vi "Signal_output_DAQ.vi"() -> ()   [LabVIEW 2013]
doc: "This example demonstrates how to continuously re-generate analog output data from a buffer in your computer's memory.\n\nRefer to your device documentation for pinouts and hardware capabilities."
uses:
  <vilib>/Utility/error.llb/DialogType.ctl
  <vilib>/DAQmx/write.llb/DAQmx Write (Analog 1D Wfm NChan NSamp).vi
  <vilib>/DAQmx/create/channels.llb/DAQmx Create Channel (AO-Voltage-Basic).vi
  <vilib>/DAQmx/configure/timing.llb/DAQmx Timing (Sample Clock).vi
  <vilib>/DAQmx/configure/trigger.llb/DAQmx Start Trigger (Digital Edge).vi
  <vilib>/DAQmx/configure/trigger.llb/DAQmx Start Trigger (Analog Edge).vi
  <vilib>/Utility/error.llb/Error Cluster From Error Code.vi
  <vilib>/DAQmx/miscellaneous.llb/DAQmx Fill In Error Info.vi
  <vilib>/ErrorRing/Error Ring.xnode
  <resource>/objmgr/daqmx.rc
panel:
  in  "sample mode":i32(ring)=10123 items=["Finite Samples"=10178, "Continuous Samples"=10123, "Hardware Timed Single Point"=12522]
  in  "Waveform settings":T1={"Tx"=0.001, "Vx_max"=0.5, "Vy_max"=0.5, "Row_N"=20, "ratio of decline"=0.3}
  in  "Trigger Type":T2(tab)
  in  "Edge":i32(ring)=10280 items=["Rising"=10280, "Falling"=10171]
  in  "Digital Trigger Source":tag
  in  "Level (V)":dbl format="%0.2f"
  in  "Hysteresis (V)":dbl
  in  "Slope":i32(ring)=10280 items=["Rising"=10280, "Falling"=10171]
  in  "Analog Trigger Source":string="APFI0"
  in  "Pause When":i32(ring)=10192 items=["High"=10192, "Low"=10214]
  in  "Pause Trigger Source":tag
  in  "Stop":bool
  out "Waveform Graph":waveform(dbl)[](graph)=[{"t0"=timestamp(0 s since 1904-01-01), "dt"=0.05, "Y"=array[353 elements]}, {"t0"=timestamp(0 s since 1904-01-01), "dt"=0.05, "Y"=array[353 elements]}]
  in  "Sample Rate":dbl=200000.0
  in  "Sample Clock Source":tag="OnboardClock"
  in  "Max Voltage":dbl=2.0
  in  "Min Voltage":dbl=-2.0
  in  "Physical Channel(s)":tag="Dev1/ao0:1"
  out "Actual Sample Rate":dbl=200000.0 format="%0.2f"
  # "Channel Settings"
  # "Output"
  # "Timing and Buffer Settings"
  # "Trigger Settings"
  # "Waveform Settings"
  # "To configure and use a start trigger you must have the necessary tab selected above.  Not all hardware supports triggering--refer to your device documentation for more info."
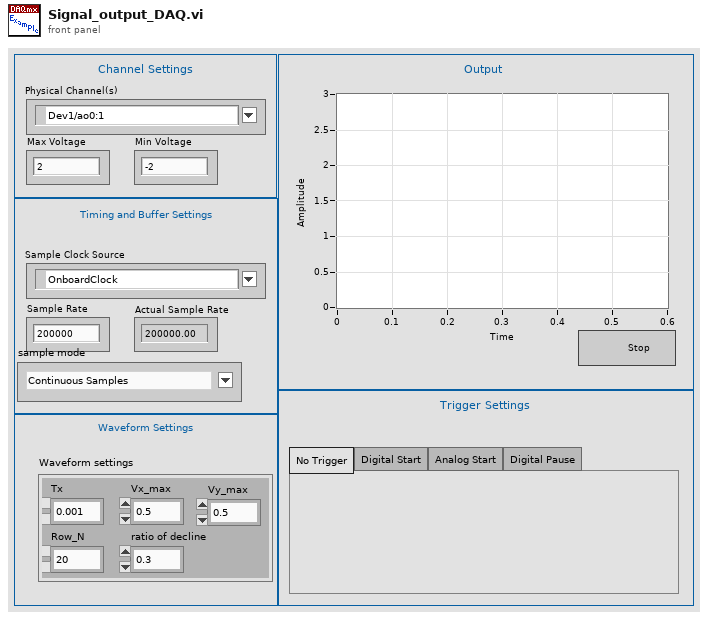
[diagram p1: front panel]
types:
  T1 = cluster{"Tx":dbl, "Vx_max":dbl, "Vy_max":dbl, "Row_N":i32, "ratio of decline":dbl}
  T2 = enum32{"No Trigger", "Digital Start", "Analog Start", "Digital Pause"}
  T3 = typedef "DialogType.ctl" = u16
  T4 = enum16{"Left Button", "Center Button", "Right Button", "Window Close"}
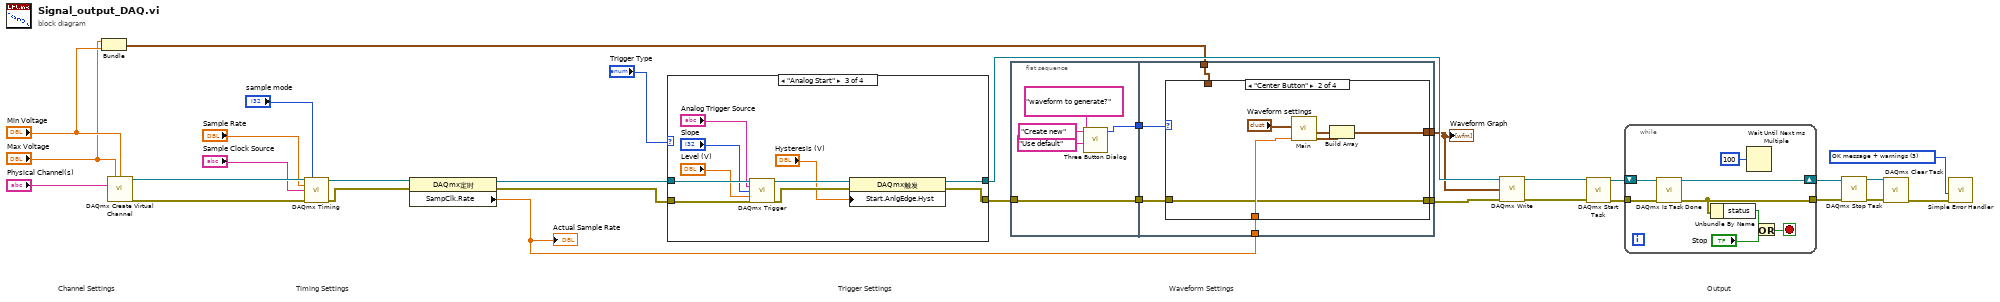
[diagram p0: block diagram]
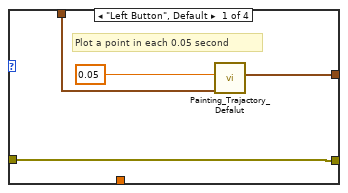
[diagram p2: hidden frame]
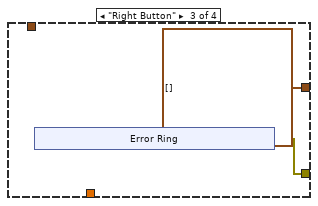
[diagram p3: hidden frame]
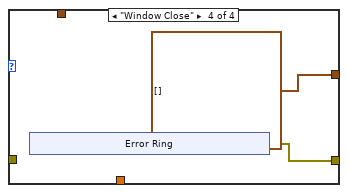
[diagram p4: hidden frame]
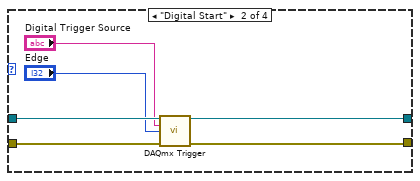
[diagram p6: hidden frame]
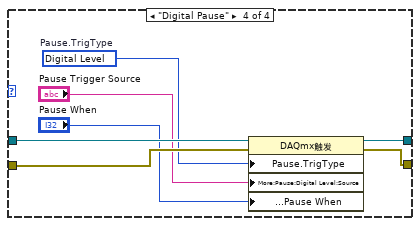
[diagram p7: hidden frame]
diagram:
  w12 = T3 3 items=["no dialog", "OK message", "continue or stop message", "OK message + warnings", "continue/stop + warnings"] ("type of dialog (OK msg:1)")
  # "Output"
  # "Trigger Settings"
  # "Waveform Settings"
  # "Timing Settings"
  # "Channel Settings"
  n1 = Bundle("Max Voltage"="Max Voltage", "Min Voltage"="Min Voltage") -> (w3:cluster{"Max Voltage":dbl, "Min Voltage":dbl})  [unwired: 1 in]
  n2 = call-poly <vilib>:"DAQmx Create Virtual Channel.vi"("maximum value"="Max Voltage", "minimum value"="Min Voltage", "physical channels"="Physical Channel(s)") -> ("task out"=w28:refnum<k21>, "error out"=w29:errorcluster)  [unwired: 11 in]
  n3 = call-poly <vilib>:"DAQmx Timing.vi"("task/channels in"=w28, "sample mode"="sample mode", "rate"="Sample Rate", "source"="Sample Clock Source", "error in"=w29) -> ("task out"=w31:refnum<k21>, "error out"=w30:errorcluster)  [unwired: 9 in]
  n4 = property class="DAQmx定时"(reference=w31, error in=w30) -> (reference out=w20:refnum<k21>, error out=w19:errorcluster, "SampClk.Rate"=w9:dbl)
  "Actual Sample Rate" <- w9
  n5 = case shown="\"Analog Start\"" "Trigger Type" {
    tunnel: w20 -> [w33 w39 w49 w56]
    tunnel: w19 -> [w32 w38 w48 w53]
    tunnel: [w33 w37 w46 w55] -> w5
    tunnel: [w32 w36 w45 w54] -> w10
    frame "No Trigger", Default {
    }
    frame "Digital Start" {
      n6 = call-poly <vilib>:"DAQmx Trigger.vi"("task/channels in"=w39, "source"="Digital Trigger Source", "edge"="Edge", "error in"=w38) -> ("task out"=w37:refnum<k21>, "error out"=w36:errorcluster)  [unwired: 10 in]
    }
    frame "Analog Start" {
      n7 = call-poly <vilib>:"DAQmx Trigger.vi"("task/channels in"=w49, "source"="Analog Trigger Source", "slope"="Slope", "level"="Level (V)", "error in"=w48) -> ("task out"=w44:refnum<k21>, "error out"=w43:errorcluster)  [unwired: 9 in]
      n8 = property class="DAQmx触发"(reference=w44, error in=w43, "Start.AnlgEdge.Hyst"="Hysteresis (V)") -> (reference out=w46:refnum<k21>, error out=w45:errorcluster)
    }
    frame "Digital Pause" {
      w52 = 10152 items=["Analog Level"=10101, "Analog Window"=10103, "Digital Level"=10152, "Digital Pattern"=10398, "None"=10230]  # Pause.TrigType
      n9 = property class="DAQmx触发"(reference=w56, error in=w53, "Pause.TrigType"=w52, "More:Pause:Digital Level:Source"="Pause Trigger Source", "More:Pause:Digital Level:Pause When"="Pause When") -> (reference out=w55:refnum<k21>, error out=w54:errorcluster)
    }
  }
  n10 = flat-sequence {
    tunnel: w10 -> [w61]
    tunnel: [w61] -> w8
    tunnel: [w60] -> w7
    tunnel: w9 -> [w67]
    tunnel: w8 -> [w65]
    tunnel: w7 -> [w66]
    tunnel: [w64] -> w6
    tunnel: [w63] -> w4
    tunnel: w3 -> [w62]
    frame #0 {
      n11 = call <vilib>:"Three Button Dialog.vi"("Center Button Text (\"No\")"="Use default" ("Center Button Text (\"No\")"), "Left Button Text (\"Yes\")"="Create new" ("Left Button Text (\"Yes\")"), "message"="waveform to generate?") -> ("Which Button?"=w60:T4)  [unwired: 8 in]
    }
    frame #1 {
      n12 = case shown="\"Center Button\"" w66 {
        tunnel: w67 -> [_ w74 _ _]
        tunnel: w65 -> [w71 w72 _ _]
        tunnel: [w71 w72 w79 w85] -> w64
        tunnel: [w70 w73 waveform(dbl)[] [] waveform(dbl)[] []] -> w63
        tunnel: w62 -> [w68 _ _ _]
        frame "Left Button", Default {
          # "Plot a point in each 0.05 second"
          n13 = call "Painting_Trajactory_Defalut.vi"("Max-Min Voltage"=w68, "dt"=0.05) -> ("Waveforms"=w70:waveform(dbl)[])  [unwired: 9 in]
        }
        frame "Center Button" {
          n14 = call "Main.vi"("Fs (Hz)"=w74, "Waveform settings"="Waveform settings") -> ("Y"=w77:waveform(dbl), "X"=w76:waveform(dbl))  [unwired: 7 in, 1 out]
          n15 = Build Array(w76, w77) -> (w73:waveform(dbl)[])
        }
        frame "Right Button" {
          n16 = xnode "Error Ring"() -> ("错误输出"=w79:errorcluster)
        }
        frame "Window Close" {
          n17 = xnode "Error Ring"() -> ("错误输出"=w85:errorcluster)
        }
      }
    }
  }
  n18 = call-poly <vilib>:"DAQmx Write.vi"("task/channels in"=w5, "data"=w4, "error in"=w6) -> ("task out"=w18:refnum<k21>, "error out"=w17:errorcluster)  [unwired: 10 in, 1 out]
  n19 = call <vilib>:"DAQmx Start Task.vi"("task/channels in"=w18, "error in"=w17) -> ("task out"=w27:refnum<k21>, "error out"=w26:errorcluster)  [unwired: 12 in]
  n20 = while {
    tunnel: w26 -> [w96]
    tunnel: [w93] -> w13
    shift-right: [w94] -> w14
    shift-left: w27 -> [w97]
    stop <- w95 stop-if-true
    n21 = call <vilib>:"DAQmx Is Task Done.vi"("task/channels in"=w97, "error in"=w96) -> ("task out"=w94:refnum<k21>, "error out"=w93:errorcluster)  [unwired: 11 in, 1 out]
    n22 = Unbundle By Name(w93) -> ("status"=w92:bool)
    n23 = Wait Until Next ms Multiple(millisecond multiple=u32 100) -> ()  [unwired: 1 out]
    n24 = Or(x=w92, y="Stop") -> (x .or. y?=w95:bool)
  }
  n25 = call <vilib>:"DAQmx Stop Task.vi"("task/channels in"=w14, "error in"=w13) -> ("task out"=w16:refnum<k21>, "error out"=w15:errorcluster)  [unwired: 12 in]
  n26 = call <vilib>:"DAQmx Clear Task.vi"("task in"=w16, "error in"=w15) -> ("error out"=w25:errorcluster)  [unwired: 13 in]
  n27 = call <vilib>:"Simple Error Handler.vi"("type of dialog (OK msg:1)"=w12, "error in (no error)"=w25) -> ()  [unwired: 3 in, 5 out]
  "Waveform Graph" <- w4
